vi "Update Channel Tree.vi"(7 "Direction to Include":T1, 8 "error in (no error)":errorcluster, 10 "Channnel Tree ref in":refnum<vi>, 11 "Channels":T3(array[cluster])) -> (0 "error out":errorcluster)   [LabVIEW 2021, in "CIF_UI.lvclass"]
uses:
  CIF_UI.lvclass
  CIFCore/Grpc/CIFCoreChannel_client/RPC Messages/cif_channelcore_Direction.ctl
  Typedef/Direction to Include.ctl
  CIF_UI.lvclass/CIF_UI.ctl
  CIFCore/Grpc/CIFCoreChannel_client/CIFCoreChannel_client.lvlib
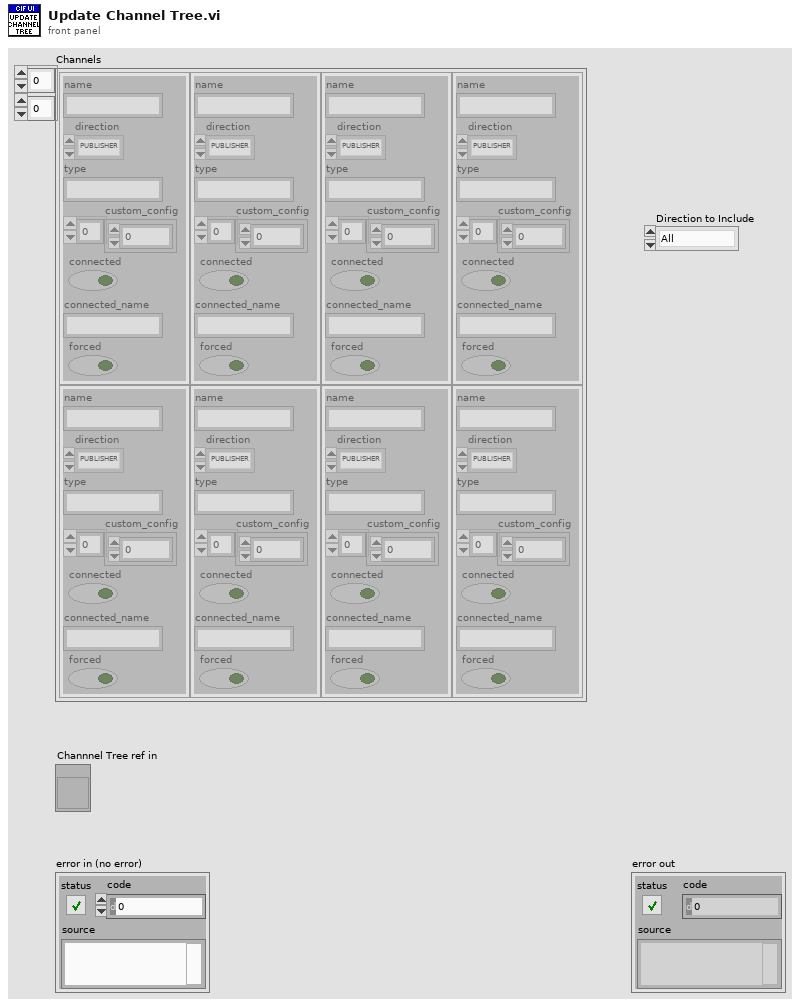
[diagram p1: front panel]
types:
  T1 = typedef "CIF_UI.lvclass/Direction to Include.ctl" = enum16{"All", "Subscriber", "Publisher"}
  T2 = typedef "CIFCoreChannel_client.lvlib/cif_channelcore_Direction.ctl" = enum32{"PUBLISHER", "SUBSCRIBER"}
  T3 = cluster{"name":string, "direction":T2, "type":string, "custom_config":u8[], "connected":bool, "connected_name":string, "forced":bool}[][]
  T4 = cluster{"name":string, "direction":T2, "type":string, "custom_config":u8[], "connected":bool, "connected_name":string, "forced":bool}
  T5 = cluster{"name":string, "direction":T2, "type":string, "custom_config":u8[], "connected":bool, "connected_name":string, "forced":bool}[]
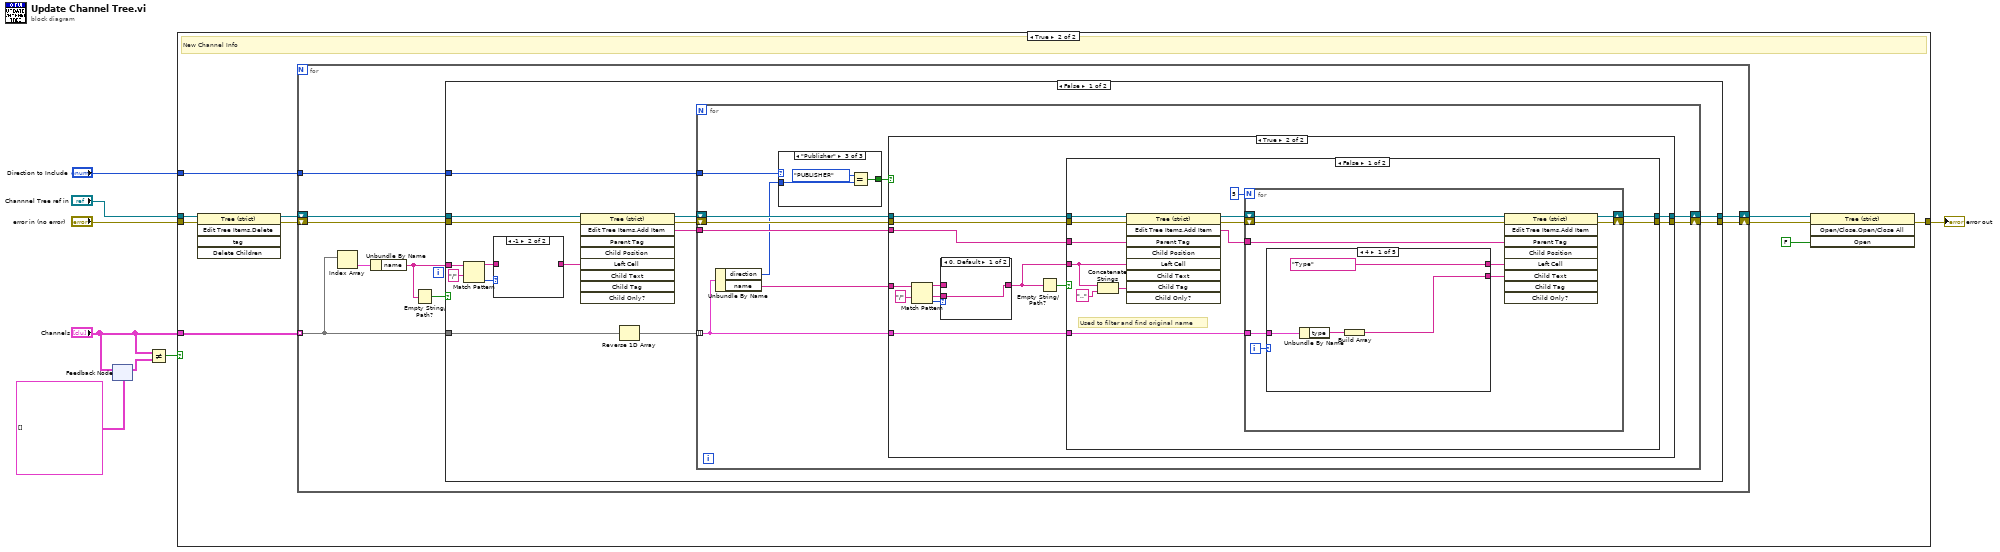
[diagram p0: block diagram]
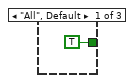
[diagram p4: hidden frame]
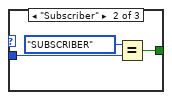
[diagram p5: hidden frame]
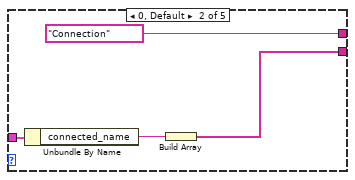
[diagram p8: hidden frame]
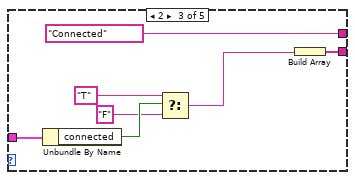
[diagram p9: hidden frame]
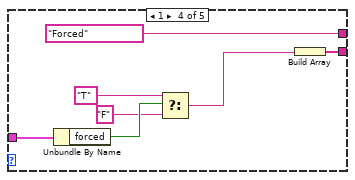
[diagram p10: hidden frame]
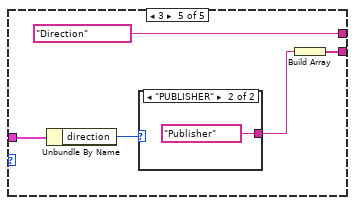
[diagram p11: hidden frame]
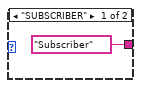
[diagram p12: hidden frame]
diagram:
  n1 = feedback-in #1("Channels") -> ()
  n2 = feedback #1(T3 [] ("Channels")) -> (w3:T3)
  n3 = Not Equal?(x="Channels", y=w3) -> (x != y?=w2:bool)
  n4 = case shown="True" w2 {
    tunnel: "error in (no error)" -> [w9 w14]
    tunnel: [w9 w13] -> w7
    tunnel: "Channnel Tree ref in" -> [_ w12]
    tunnel: "Channels" -> [_ w11]
    tunnel: "Direction to Include" -> [_ w10]
    frame False {
      # "No updates"
    }
    frame True {
      # "New Channel Info"
      n5 = invoke class="Tree (strict)" method="Edit Tree Items.Delete"(reference=w12, error in=w14) -> (reference out=w18:refnum<vi>, error out=w19:errorcluster)  [unwired: 3 in, 3 out]
      n6 = for {
        shift-right: [w27] -> w17
        shift-left: w18 -> [w26]
        tunnel: w11 -> [w24] mode=indexing
        tunnel: w10 -> [w22]
        shift-right: [w28] -> w16
        shift-left: w19 -> [w25]
        n7 = Index Array(array=w24) -> (element=w23:T4)  [unwired: 1 in]
        n8 = Unbundle By Name(w23) -> ("name"=w21:string)
        n9 = Empty String/Path?(string/path=w21) -> (empty?=w20:bool)
        n10 = case shown="False" w20 {
          tunnel: [w43 w132] -> w28
          tunnel: [w42 w133] -> w27
          tunnel: w26 -> [w41 w133]
          tunnel: w25 -> [w40 w132]
          tunnel: w24 -> [w39 _]
          tunnel: w22 -> [w38 _]
          tunnel: w21 -> [w29 _]
          frame False {
            n11 = Match Pattern(string=w29, regular expression="/") -> (before substring=w32:string, offset past match=w33:i32)  [unwired: 1 in, 2 out]
            n12 = case shown="-1" w33 {
              tunnel: w32 -> [w44 _]
              tunnel: [w44 _] -> w31
              frame 0, Default {
              }
              frame -1 {
              }
            }
            n13 = invoke class="Tree (strict)" method="Edit Tree Items.Add Item"(reference=w41, error in=w40, "Left Cell"=w31) -> (reference out=w37:refnum<vi>, error out=w36:errorcluster, "Edit Tree Items:Add Item"=w35:string)  [unwired: 6 in, 6 out]
            n14 = Reverse 1D Array(array=w39) -> (reversed array=w30:T5)
            n15 = for {
              tunnel: w35 -> [w52]
              shift-right: [w50] -> w42
              shift-left: w37 -> [w54]
              shift-right: [w51] -> w43
              shift-left: w36 -> [w53]
              tunnel: w30 -> [w49] mode=indexing
              tunnel: w38 -> [w45]
              n16 = Unbundle By Name(w49) -> ("direction"=w46:T2, "name"=w48:string)
              n17 = case shown="\"Publisher\"" w45 {
                tunnel: [TRUE w58 w61] -> w47
                tunnel: w46 -> [_ w56 w59]
                frame "All", Default {
                }
                frame "Subscriber" {
                  n18 = Equal?(x=cif_channelcore_Direction."SUBSCRIBER" ("direction"), y=w56) -> (x = y?=w58:bool)
                }
                frame "Publisher" {
                  n19 = Equal?(x=cif_channelcore_Direction."PUBLISHER" ("direction"), y=w59) -> (x = y?=w61:bool)
                }
              }
              n20 = case shown="True" w47 {
                tunnel: w54 -> [w63 w76]
                tunnel: w53 -> [w62 w75]
                tunnel: w52 -> [_ w74]
                tunnel: [w62 w73] -> w51
                tunnel: [w63 w72] -> w50
                tunnel: w49 -> [_ w71]
                tunnel: w48 -> [_ w67]
                frame False {
                }
                frame True {
                  n21 = Match Pattern(string=w67, regular expression="/") -> (before substring=w65:string, after substring=w66:string, offset past match=w69:i32)  [unwired: 1 in, 1 out]
                  n22 = case shown="0, Default" w69 {
                    tunnel: [w77 w78] -> w64
                    tunnel: w66 -> [w77 _]
                    tunnel: w65 -> [_ w78]
                    frame 0, Default {
                    }
                    frame -1 {
                    }
                  }
                  n23 = Empty String/Path?(string/path=w64) -> (empty?=w70:bool)
                  n24 = case shown="False" w70 {
                    tunnel: w76 -> [w91 w131]
                    tunnel: w75 -> [w90 w130]
                    tunnel: w74 -> [w87 _]
                    tunnel: [w85 w130] -> w73
                    tunnel: [w84 w131] -> w72
                    tunnel: w71 -> [w83 _]
                    tunnel: w64 -> [w81 _]
                    frame False {
                      # "Used to filter and find original name"
                      n25 = Concatenate Strings(w81, "..") -> (w80:string)
                      n26 = invoke class="Tree (strict)" method="Edit Tree Items.Add Item"(reference=w91, error in=w90, "Parent Tag"=w87, "Left Cell"=w81, "Child Tag"=w80) -> (reference out=w89:refnum<vi>, error out=w88:errorcluster, "Edit Tree Items:Add Item"=w86:string)  [unwired: 4 in, 6 out]
                      n27 = for {
                        N: 5 -> [_]
                        tunnel: w86 -> [w98]
                        shift-right: [w96] -> w84
                        shift-left: w89 -> [w100]
                        shift-right: [w97] -> w85
                        shift-left: w88 -> [w99]
                        tunnel: w83 -> [w95]
                        i -> [w94]
                        n28 = case shown="4" w94 {
                          tunnel: w95 -> [w104 w108 w115 w122 w127]
                          tunnel: [w102 w106 w114 w121 w126] -> w93
                          tunnel: ["Type" "Connection" "Connected" "Forced" "Direction"] -> w92
                          frame 4 {
                            n29 = Unbundle By Name(w104) -> ("type"=w103:string)
                            n30 = Build Array(w103) -> (w102:string[])
                          }
                          frame 0, Default {
                            n31 = Unbundle By Name(w108) -> ("connected_name"=w107:string)
                            n32 = Build Array(w107) -> (w106:string[])
                          }
                          frame 2 {
                            n33 = Unbundle By Name(w115) -> ("connected"=w111:bool)
                            n34 = Select(t="T", s=w111, f="F") -> (s? t:f=w110:string)
                            n35 = Build Array(w110) -> (w114:string[])
                          }
                          frame 1 {
                            n36 = Unbundle By Name(w122) -> ("forced"=w118:bool)
                            n37 = Select(t="T", s=w118, f="F") -> (s? t:f=w117:string)
                            n38 = Build Array(w117) -> (w121:string[])
                          }
                          frame 3 {
                            n39 = Unbundle By Name(w127) -> ("direction"=w124:T2)
                            n40 = case shown="\"PUBLISHER\"" w124 {
                              tunnel: ["Subscriber" "Publisher"] -> w123
                              frame "SUBSCRIBER" {
                              }
                              frame "PUBLISHER" {
                              }
                            }
                            n41 = Build Array(w123) -> (w126:string[])
                          }
                        }
                        n42 = invoke class="Tree (strict)" method="Edit Tree Items.Add Item"(reference=w100, error in=w99, "Parent Tag"=w98, "Left Cell"=w92, "Child Text"=w93) -> (reference out=w96:refnum<vi>, error out=w97:errorcluster)  [unwired: 4 in, 7 out]
                      }
                    }
                    frame True {
                    }
                  }
                }
              }
            }
          }
          frame True {
          }
        }
      }
      n43 = invoke class="Tree (strict)" method="Open/Close.Open/Close All"(reference=w17, error in=w16, "Open"=FALSE ("Open?")) -> (error out=w13:errorcluster)  [unwired: 1 in, 3 out]
    }
  }
  "error out" <- w7
